vi "MessageConverterProxy.vi"(5 "package_templatemessage_type":T1, 11 "serialized_templatemessage":T1) -> (3 "package_templatemessage":T1)   [LabVIEW 2019, in "Service Template.lvlib"]
uses:
  Service Template.lvlib
  package_templatemessage.ctl
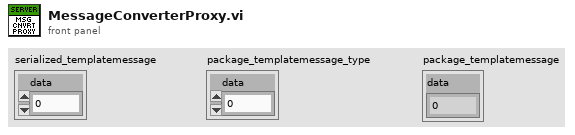
[diagram p1: front panel]
types:
  T1 = typedef "Service Template.lvlib/package_templatemessage.ctl" = cluster{"data":sgl}
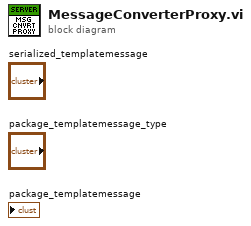
[diagram p0: block diagram]
diagram:
